vi "niRFUtil FTW Generate No Response.vi"(2 "Minimum Selectivity (dB)":dbl=70.0 format="%.2f", 3 "df (Hz)":dbl format="%^.2e", 4 "Bandwidth (Hz)":T3 format="%^.3e", 5 "Center Frequency (Hz)":dbl format="%^.2e") -> (0 "-ENBW (dB-Hz)":sgl format="%.2f", 1 "Filter Power Response":T1 {"y" min=0 max=127 format="%.2f"; "dx" format="%^.2e"; "x0" format="%^.2e"})   [LabVIEW 2015, in "niRFUtil.lvlib"]
doc: "(c) Copyright 2006, National Instruments, Inc. This VI may not be duplicated, sold, or distributed without written consent from National Instruments."
uses:
  niRFUtil.lvlib
  Includes/niRFUtil INC RBW Filter Bandwidth.ctl
  Includes/niRFUtil INC Real Waveform.ctl
  Includes/niRFUtil INC Real Array.ctl
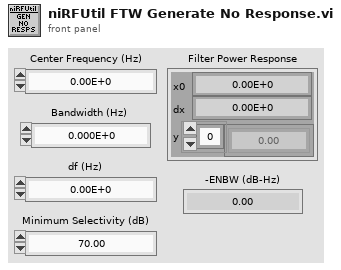
[diagram p1: front panel]
types:
  T1 = typedef "niRFUtil.lvlib/niRFUtil INC Real Waveform.ctl" = cluster{"x0":dbl, "dx":dbl, "y":T2}
  T2 = typedef "niRFUtil.lvlib/niRFUtil INC Real Array.ctl" = sgl[]
  T3 = typedef "niRFUtil.lvlib/niRFUtil INC RBW Filter Bandwidth.ctl" = dbl
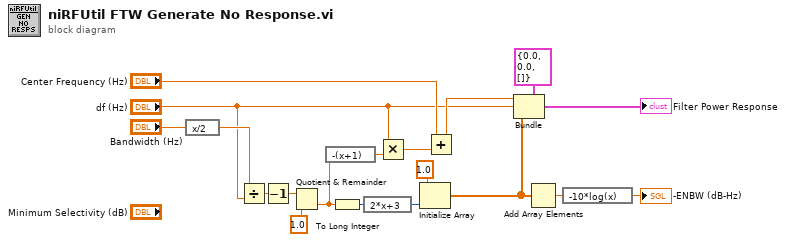
[diagram p0: block diagram]
diagram:
  n1 = expression code="x/2"("Bandwidth (Hz)") -> (w9:T3)
  n2 = Divide(x=w9, y="df (Hz)") -> (x/y=w15:T3)
  n3 = Decrement(x=w15) -> (x-1=w8:T3)
  n4 = Quotient & Remainder(x=w8, y=1.0) -> (floor(x/y)=w13:T3)  [unwired: 1 out]
  n5 = expression code="-(x+1)"(w13) -> (w12:T3)
  n6 = To Long Integer(number=w13) -> (32bit integer=w18:i32)
  n7 = expression code="2*x+3"(w18) -> (w17:i32)
  n8 = Multiply(x="df (Hz)", y=w12) -> (x*y=w11:T3)
  n9 = Initialize Array(sgl 1.0 ("element"), w17) -> (w2:sgl[])
  n10 = Add(x="Center Frequency (Hz)", y=w11) -> (x+y=w10:T3)
  n11 = Bundle(cluster=T1 {"x0"=0.0, "dx"=0.0, "y"=[]} ("Filter Power Response"), "x0"=w10, "dx"="df (Hz)", "y"=w2) -> (→"Filter Power Response":T1)
  n12 = Add Array Elements(numeric array=w2) -> (sum=w3:sgl)
  n13 = expression code="-10*log(x)"(w3) -> (→"-ENBW (dB-Hz)":sgl)
